vi "View AI param.vi"(7 "ActivateAIView":bool, 9 "AIP":T1, 10 "AI_State":T3[](array[typedef]), 11 "AITable":dbl[](array[numeric]) format="%#.0f") -> (2 "Reread out":bool)   [LabVIEW 2019, in "Inputs.lvlib"]
uses:
  Inputs.lvlib
  Ctl/Parameter State.ctl
  Ctl/AI.ctl
  Ctl/AI short.ctl
  Database/Progress.vi
  Database/PostgreSQL.lvlib
panel:
  out "fcode_full":string[](array[string])=["H1.EB2.1.BT1", "H1.EB2.1.BT3", "H1.EB2.21.BT1", "H1.EB2.22.BT1", "H1.EB2.23.BT1", "H1.EB2.2.BT3", "H1.EB2.BP1", "H1.EB2.EP1.BF1", "H1.EB2.EP1.BT1", "H1.EB2.EP1.BT2", "H1.EB2.QN1", "H1.EP.BP1", "H1.GM2.1.BP1", "H1.GM2.1.HT1.BC1", "H1.GM2.1.HT1.BT1", "H1.GM2.1.QN1", "H1.GM2.2.BP1", "H1.GM2.2.QN1", "H1.GM2.2.QN2", "H1.GM2.2.QN3", "H1.HW2.BT1", "H1.HW2.BT2", "H1.HW2.BT3", "H1.HW2.BT4"]
  out "Names":string[](array[string])=["температура нагревателя", "температура газа после ступени", "температура нагревателя", "температура нагревателя", "температура нагревателя", "температура газа после ступени", "давление газа перед нагревателем", "расход охлаждающей воды", "температура на входе", "температура на выходе", "регулятор расхода азота/тех газа", "давление охлаждающей воды на входе в теплообменник", "давление газа перед дозатором", "ток нагревателя", "температура нагревателя", "регулятор расхода азота/водорода (метана)", "давление газа перед дозатором", "регулятор расхода водорода (метана)", "регулятор природного газа", "дозатор жидкостный", "температура газа на входе в смеситель", "температура стенки смесителя 100 мм", "температура стенки смесителя 200 мм", "температура стенки смесителя на вводе CH4"]
  out "units":string[](array[string])
  out "AI progress":i32(slide) scale=0.0..100.0
  in  "Reread":bool
  in  "n_elem":i32(c297)
  out "AI_9":dbl format="%#.1f"
  out "AI_10":dbl format="%#.1f"
  out "AI_5":dbl format="%#.1f"
  out "AI_6":dbl format="%#.1f"
  out "AI_7":dbl format="%#.1f"
  out "AI_8":dbl format="%#.1f"
  out "AI_3":dbl format="%#.1f"
  out "AI_4":dbl format="%#.1f"
  out "AI_2":dbl format="%#.1f"
  out "AI_1":dbl format="%#.1f"
  out "n param":i32
  out "Parameters":dbl[][](array[numeric])=[[1.0, 0.0, 1000.0, 2.0, 0.0, 0.0, 2.0, 20.0, 100.0, nan, 250.0, 250.0, 2.0, 1.0, 10.0, 0.0, 65535.0, 0.0, 250.0, 1.0, 4.0], [1.0, 0.0, 1000.0, 2.0, 0.0, 0.0, 2.0, 20.0, 150.0, nan, 250.0, 250.0, 2.0, 1.0, 11.0, 0.0, 65535.0, 0.0, 250.0, 0.0, 4.0], [1.0, 0.0, 1000.0, 2.0, 0.0, 0.0, 2.0, 3.0, 7.0, 8.0, 10.0, 10.0, 2.0, 0.1, 1.0, 0.0, 65535.0, 0.0, 10.0, 0.0, 2.0], [1.0, 0.0, 1000.0, 2.0, 0.0, 0.0, 1.5, 2.5, 6.0, 7.0, 10.0, 10.0, 2.0, 0.1, 2.0, 0.0, 65535.0, 0.0, 10.0, 0.0, 3.0], [1.0, 0.0, 1000.0, 2.0, 0.0, 0.0, 2.0, 2.5, 6.0, 7.0, 10.0, 10.0, 2.0, 0.1, 3.0, 0.0, 65535.0, 0.0, 10.0, 1.0, 2.0], [1.0, 0.0, 1000.0, 2.0, 0.0, 0.0, 1.5, 2.0, 4.0, 5.0, 10.0, 10.0, 2.0, 0.1, 4.0, 0.0, 65535.0, 0.0, 10.0, 1.0, 3.0], [1.0, 0.0, 1000.0, 2.0, 0.0, 0.0, 3.0, 4.0, 8.0, 9.0, 10.0, 10.0, 2.0, 0.1, 5.0, 0.0, 65535.0, 0.0, 100.0, 1.0, 7.0], [1.0, 0.0, 1000.0, 2.0, 0.0, 0.0, 4.0, 8.0, nan, nan, 100.0, 100.0, 2.0, 1.0, 6.0, 0.0, 65535.0, 0.0, 100.0, 0.0, 0.0], [1.0, 0.0, 1000.0, 2.0, 0.0, 0.0, nan, nan, nan, nan, 100.0, 100.0, 2.0, 1.0, 7.0, 0.0, 65535.0, 0.0, 100.0, 0.0, 1.0], [1.0, 0.0, 1000.0, 2.0, 0.0, 0.0, nan, nan, nan, nan, 100.0, 100.0, 2.0, 1.0, 8.0, 0.0, 65535.0, 0.0, 100.0, 1.0, 0.0], [1.0, 0.0, 1000.0, 2.0, 0.0, 0.0, 10.0, 15.0, 45.0, 50.0, 100.0, 100.0, 2.0, 1.0, 9.0, 0.0, 65535.0, 0.0, 100.0, 1.0, 1.0]]
  # "instrument_range_max"
  # "instrument_max_offset"
  # "instrument_min_offset"
  # "instrument_range_min"
  # "process_range_min"
  # "process_low_acd"
  # "d"
  # "input_register_min"
  # "input_register_max"
  # "input_pv_min"
  # "input_pv_max"
  # "control_channel_num"
  # "process_range_max"
  # "instrument_offset"
  # "process_high_acd"
  # "process_high_alr"
  # "instrument_gain"
  # "process_low_alr"
  # "module_num"
  # "time_const"
  # "Analog parameters"
  # "Description of analog parameters"
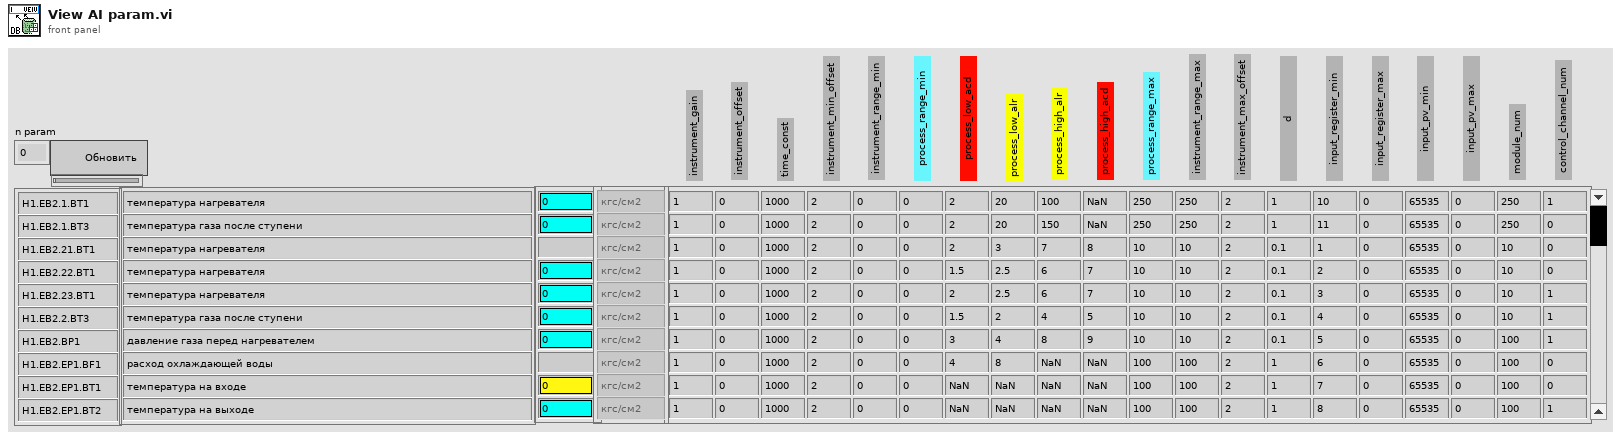
[diagram p1: front panel]
types:
  T1 = typedef "Inputs.lvlib/AI.ctl" = cluster{"AI_defs":T2, "modified":refnum<data-value>, "AIP":refnum<data-value>, "AINames":refnum<data-value>}
  T2 = typedef "Inputs.lvlib/AI short.ctl" = cluster{"AI":dbl[], "AIState":T3[], "AIALRState":errorcluster[]}
  T3 = typedef "Inputs.lvlib/Parameter State.ctl" = cluster{"code":i32, "visible":bool, "color":u32, "source":string}
  T4 = enum32{"Invalid", "Standard", "Closed", "Hidden", "Minimized", "Maximized"}
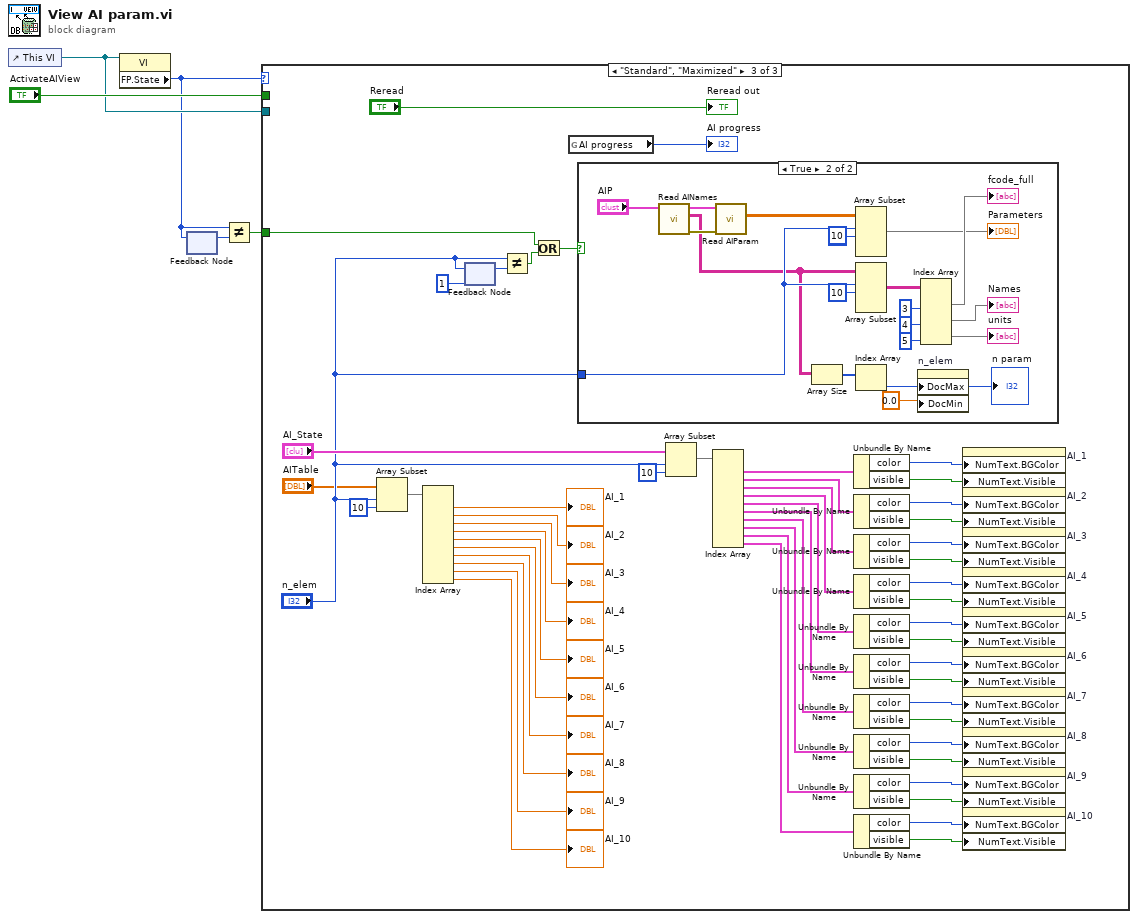
[diagram p0: block diagram]
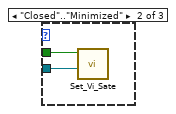
[diagram p3: hidden frame]
diagram:
  n1 = control-ref of="This VI"() -> (w4:refnum<vi>)
  n2 = property class="VI"(reference=w4) -> ("FP.State"=w1:T4)  [unwired: 1 in, 2 out]
  n3 = feedback #1() -> (w3:T4)  [unwired: 1 in]
  n4 = feedback-in #1(w1) -> ()
  n5 = Not Equal?(x=w1, y=w3) -> (x != y?=w2:bool)
  n6 = case shown="\"Standard\", \"Maximized\"" w1 {
    tunnel: "ActivateAIView" -> [_ w6 _]
    tunnel: w4 -> [_ w7 _]
    tunnel: w2 -> [_ _ w14]
    frame "Invalid", Default {
    }
    frame "Closed".."Minimized" {
      n7 = call "Set_Vi_Sate.vi"("VI"=w7, "Activate (F)"=w6) -> ()  [unwired: 9 in, 1 out]
    }
    frame "Standard", "Maximized" {
      n8 = Array Subset(array="AITable", index="n_elem", length=10) -> (w9:dbl[])
      n9 = Index Array(array=w9) -> (element #1=→"AI_1":dbl, element #2=→"AI_2":dbl, element #3=→"AI_3":dbl, element #4=→"AI_4":dbl, element #5=→"AI_5":dbl, element #6=→"AI_6":dbl, element #7=→"AI_7":dbl, element #8=→"AI_8":dbl, element #9=→"AI_9":dbl, element #10=→"AI_10":dbl)  [unwired: 10 in]
      n10 = feedback #2(1 ("n_elem")) -> (w18:i32)
      n11 = feedback-in #2("n_elem") -> ()
      n12 = Not Equal?(x="n_elem", y=w18) -> (x != y?=w17:bool)
      n13 = Or(x=w14, y=w17) -> (x .or. y?=w15:bool)
      n14 = global read "Progress.vi" "AI progress"() -> (→"AI progress":i32)
      n15 = case shown="True" w15 {
        tunnel: "n_elem" -> [_ w76]
        frame False {
        }
        frame True {
          (unwired) 10 ("length")
          n16 = call "Read AINames.vi"("AI in"="AIP") -> ("error out"=w66:errorcluster, "AINames"=w63:string[][], "AI out"=w65:T1)  [unwired: 8 in]
          n17 = call "Read AIParam.vi"("error in (no error)"=w66, "AI in"=w65) -> ("AIParam"=w62:dbl[][])  [unwired: 7 in, 2 out]
          n18 = Array Size(array=w63) -> (size(s)=w73:i32[])
          n19 = Array Subset(array=w62, index (row)=w76, length (row)=10 ("length")) -> (→"Parameters":dbl[][])  [unwired: 2 in]
          n20 = Array Subset(array=w63, index (row)=w76, length (row)=10 ("length")) -> (w80:string[][])  [unwired: 2 in]
          n21 = Index Array(array=w73) -> (element=w71:i32)  [unwired: 1 in]
          "n param" <- w71
          n22 = property on="n_elem" class="Scroll (strict)"("DocMax"=w71, "DocMin"=0.0 ("Data Entry Limits:Minimum")) -> ()  [unwired: 2 in, 2 out]
          n23 = Index Array(array=w80, index (col) #1=3 ("disabled index (col)"), index (col) #2=4 ("disabled index (col)"), index (col) #3=5 ("index (col)")) -> (element #1=→"fcode_full":string[], element #2=→"Names":string[], element #3=→"units":string[])  [unwired: 3 in]
        }
      }
      n24 = Array Subset(array="AI_State", index="n_elem", length=10) -> (w8:T3[])
      n25 = Index Array(array=w8) -> (element #1=w23:T3, element #2=w24:T3, element #3=w25:T3, element #4=w44:T3, element #5=w45:T3, element #6=w46:T3, element #7=w47:T3, element #8=w48:T3, element #9=w49:T3, element #10=w50:T3)  [unwired: 10 in]
      n26 = Unbundle By Name(w23) -> ("color"=w12:u32, "visible"=w19:bool)
      n27 = Unbundle By Name(w24) -> ("color"=w26:u32, "visible"=w27:bool)
      n28 = Unbundle By Name(w25) -> ("color"=w28:u32, "visible"=w29:bool)
      n29 = Unbundle By Name(w44) -> ("color"=w30:u32, "visible"=w31:bool)
      n30 = Unbundle By Name(w45) -> ("color"=w32:u32, "visible"=w33:bool)
      n31 = Unbundle By Name(w46) -> ("color"=w34:u32, "visible"=w35:bool)
      n32 = Unbundle By Name(w47) -> ("color"=w36:u32, "visible"=w37:bool)
      n33 = Unbundle By Name(w48) -> ("color"=w38:u32, "visible"=w39:bool)
      n34 = Unbundle By Name(w49) -> ("color"=w40:u32, "visible"=w41:bool)
      n35 = Unbundle By Name(w50) -> ("color"=w42:u32, "visible"=w43:bool)
      n36 = property on="AI_1" class="DigNum (strict)"("NumText.BGColor"=w12, "NumText.Visible"=w19) -> ()  [unwired: 2 in, 2 out]
      n37 = property on="AI_2" class="DigNum (strict)"("NumText.BGColor"=w26, "NumText.Visible"=w27) -> ()  [unwired: 2 in, 2 out]
      n38 = property on="AI_3" class="DigNum (strict)"("NumText.BGColor"=w28, "NumText.Visible"=w29) -> ()  [unwired: 2 in, 2 out]
      n39 = property on="AI_4" class="DigNum (strict)"("NumText.BGColor"=w30, "NumText.Visible"=w31) -> ()  [unwired: 2 in, 2 out]
      n40 = property on="AI_5" class="DigNum (strict)"("NumText.BGColor"=w32, "NumText.Visible"=w33) -> ()  [unwired: 2 in, 2 out]
      n41 = property on="AI_6" class="DigNum (strict)"("NumText.BGColor"=w34, "NumText.Visible"=w35) -> ()  [unwired: 2 in, 2 out]
      n42 = property on="AI_7" class="DigNum (strict)"("NumText.BGColor"=w36, "NumText.Visible"=w37) -> ()  [unwired: 2 in, 2 out]
      n43 = property on="AI_8" class="DigNum (strict)"("NumText.BGColor"=w38, "NumText.Visible"=w39) -> ()  [unwired: 2 in, 2 out]
      n44 = property on="AI_9" class="DigNum (strict)"("NumText.BGColor"=w40, "NumText.Visible"=w41) -> ()  [unwired: 2 in, 2 out]
      n45 = property on="AI_10" class="DigNum (strict)"("NumText.BGColor"=w42, "NumText.Visible"=w43) -> ()  [unwired: 2 in, 2 out]
      "Reread out" <- "Reread"
    }
  }
